vi "Dispatch Worker Mode Example(Async).vi"() -> ()   [LabVIEW 2014]
uses:
  user.lib/_NEVSTOP/JKI State Machine ++/_Support/JKISMQ/_JKISMQFGV.vi
  user.lib/_NEVSTOP/JKI State Machine ++/JKI-State-Machine-Plus.lvlib
panel:
  in  "Macro: Exit -@ Worker":bool
  in  "DoSth: DoA -@ Worker":bool
  in  "Name(\"\" to use uuid)":string="Event JKISM"
  out "State History":string
  in  "DoSth: DoA -> Worker":bool
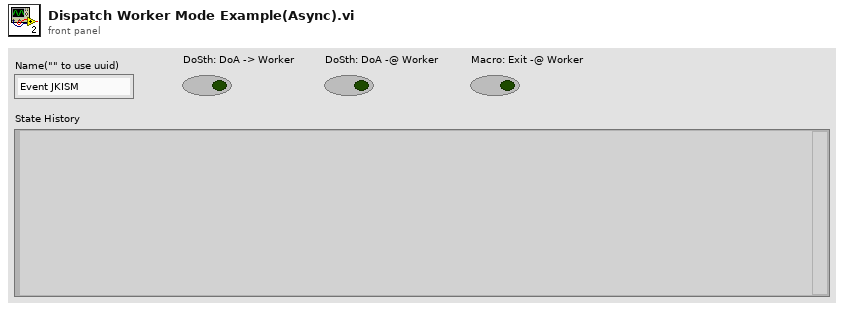
[diagram p1: front panel]
types:
  T1 = enum32{"Invalid", "Standard", "Closed", "Hidden", "Minimized", "Maximized"}
  T2 = enum32{"invalid app kind", "Development System", "Run Time System", "Student Edition", "Embedded LabVIEW", "Evaluation", "Custom"}
  T3 = cluster{"Core":cluster{"Current VI Reference":refnum<vi>, "Close Panel on Exit?":bool}, "Your Boolean data":bool, "Your string data":string}
  T4 = cluster{"Current VI Reference":refnum<vi>, "Close Panel on Exit?":bool}
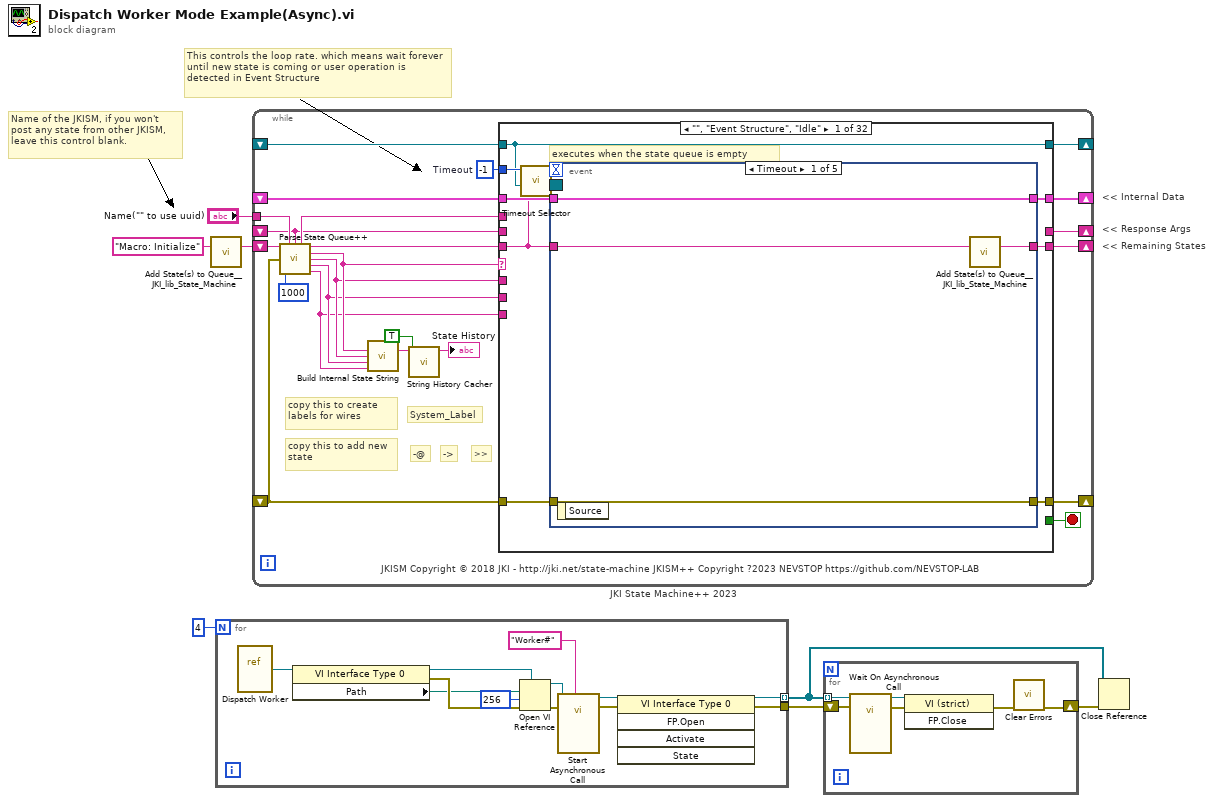
[diagram p0: block diagram]
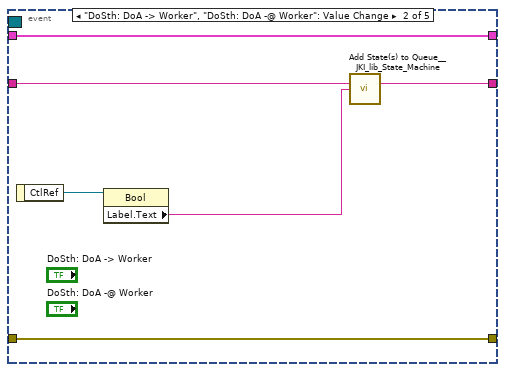
[diagram p2: hidden frame]
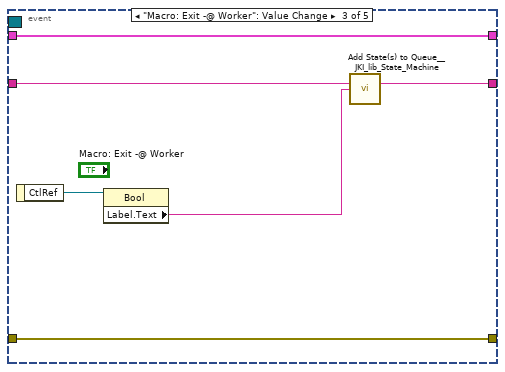
[diagram p3: hidden frame]
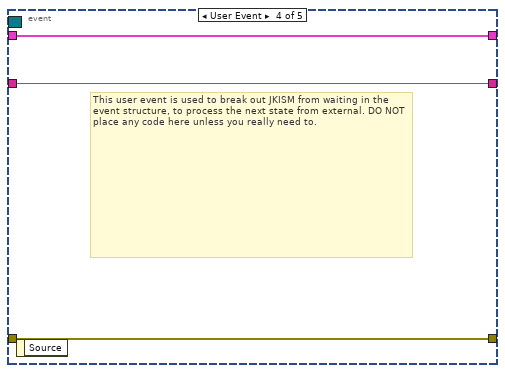
[diagram p4: hidden frame]
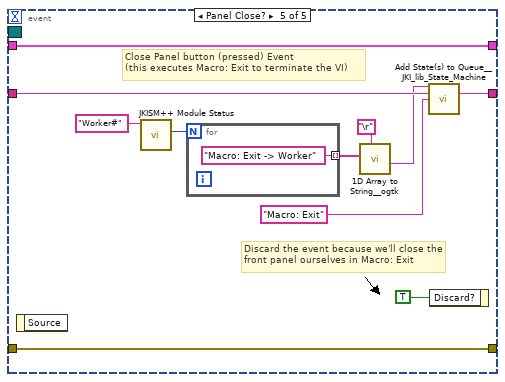
[diagram p5: hidden frame]
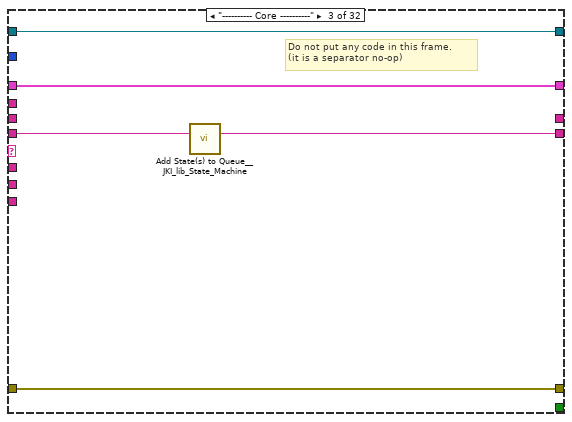
[diagram p7: hidden frame]
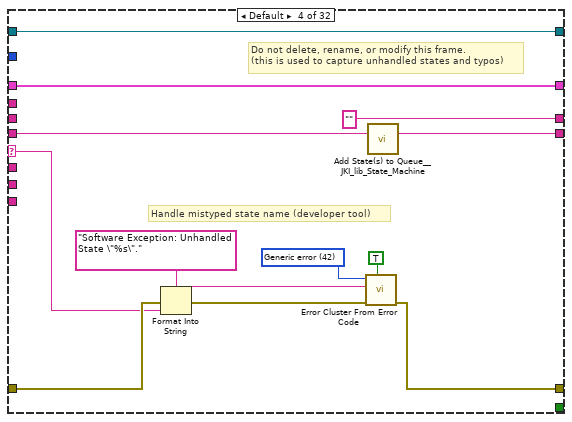
[diagram p8: hidden frame]
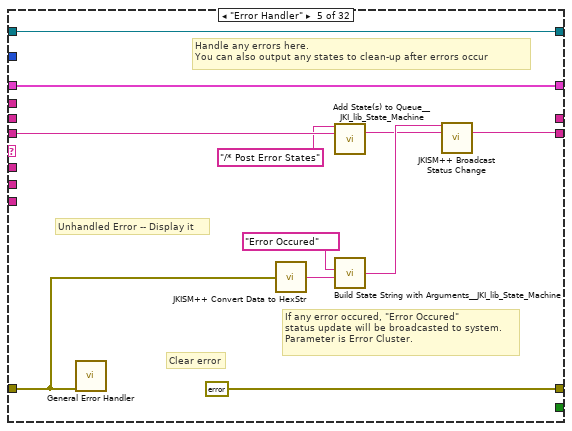
[diagram p9: hidden frame]
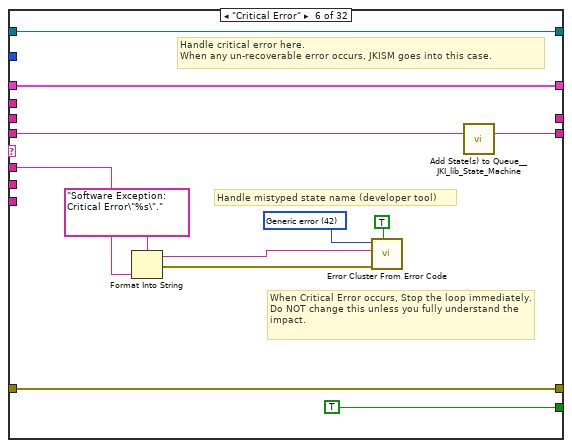
[diagram p10: hidden frame]
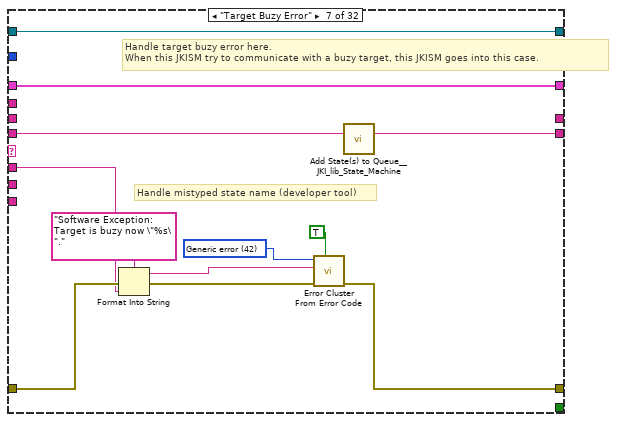
[diagram p11: hidden frame]
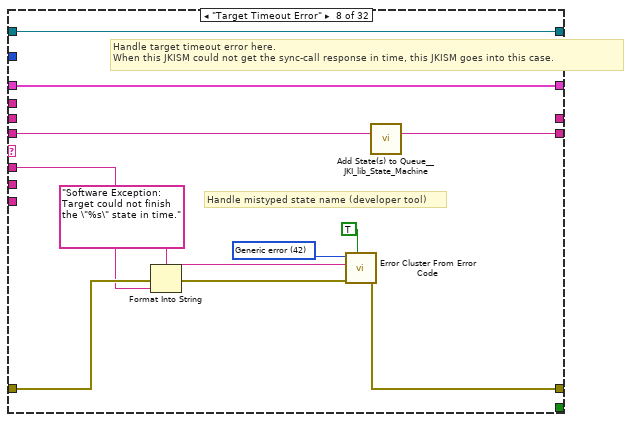
[diagram p12: hidden frame]
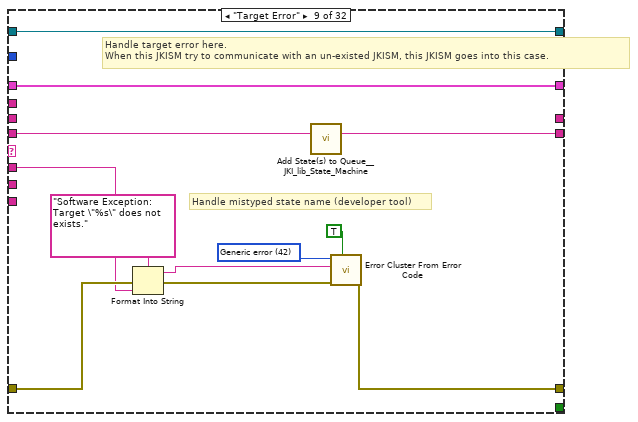
[diagram p13: hidden frame]
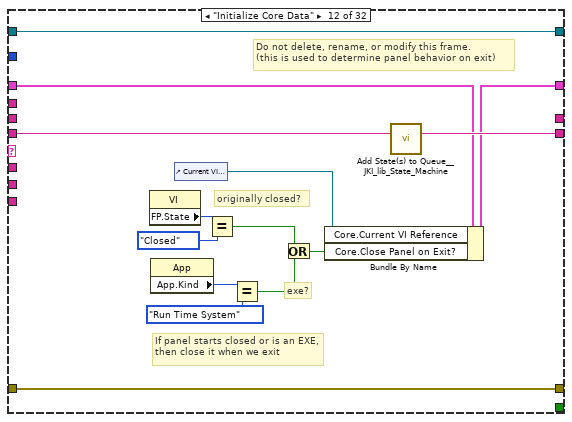
[diagram p16: hidden frame]
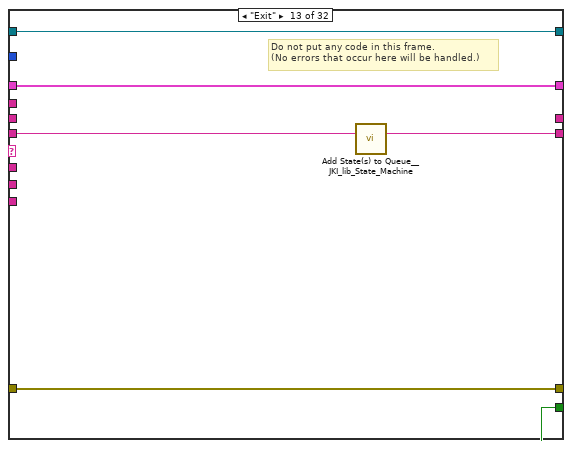
[diagram p17: hidden frame]
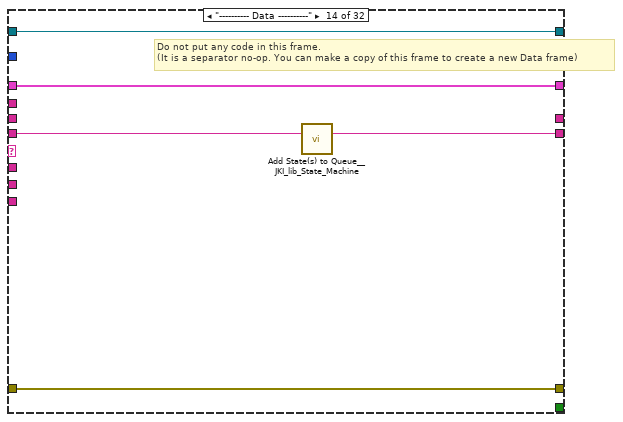
[diagram p18: hidden frame]
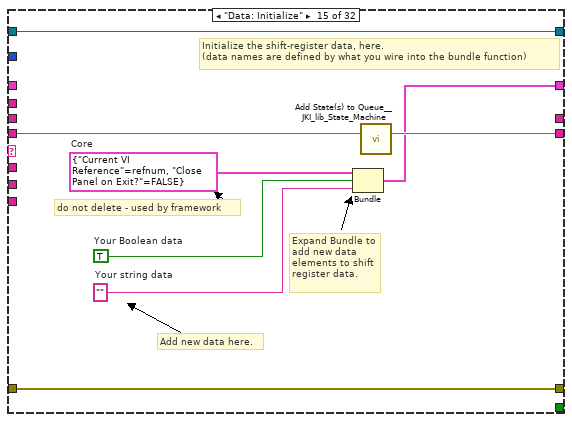
[diagram p19: hidden frame]
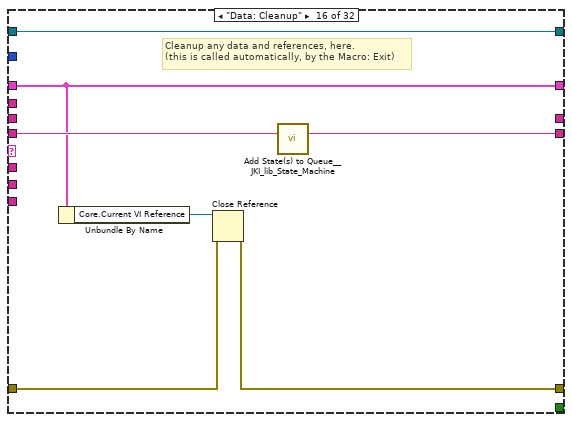
[diagram p20: hidden frame]
diagram:
  # "Name of the JKISM, if you won't post any state from other JKISM,  leave this control blank."
  # "This controls the loop rate. which means wait forever until new state is coming or user operation is detected in Event Structure"
  # "<< Internal Data"
  # "<< Response Args"
  # "<< Remaining States"
  n1 = call <vilib>:"Add State(s) to Queue__JKI_lib_State_Machine.vi"("State(s) in (\"\")"="Macro: Initialize") -> ("States Out"=w7:string)  [unwired: 14 in]
  n2 = for {
    N: 4 -> [_]
    tunnel: [w9] -> w4
    tunnel: [w10] -> w1 mode=indexing
    n3 = vi-ref "Dispatch Worker.vi"() -> (w13:refnum<vi>)
    n4 = property class="VI Interface Type 0"(reference=w13) -> (reference out=w17:refnum<vi>, error out=w15:errorcluster, "Path"=w14:path)  [unwired: 1 in]
    n5 = Open VI Reference(type specifier VI Refnum (for type only)=w17, vi path=w14, options=256, error in (no error)=w15) -> (vi reference=w16:refnum<vi>, error out=w12:errorcluster)  [unwired: 2 in]
    n6 = call-by-ref "Start Asynchronous Call"(reference=w16, error in=w12, "Name(\"\" to use uuid)"="Worker#" ("Name(\"\" to use uuid)")) -> (reference out=w11:refnum<vi>, error out=w8:errorcluster)  [unwired: 11 in]
    n7 = invoke class="VI Interface Type 0" method="FP.Open"(reference=w11, error in=w8) -> (reference out=w10:refnum<vi>, error out=w9:errorcluster)  [unwired: 3 in, 3 out]
  }
  n8 = while "JKI State Machine++ 2023" {
    shift-right: [w37] -> _
    shift-left: _ -> [w36]
    shift-right: [w40] -> _
    shift-left: _ -> [w34]
    shift-right: [w39] -> _
    shift-left: w7 -> [w41]
    tunnel: "Name(\"\" to use uuid)" -> [w29]
    shift-right: [w32] -> _
    shift-left: _ -> [w21]
    shift-right: [w31] -> _
    shift-left: _ -> [w30]
    stop <- w38 stop-if-true
    w35 = -1  # Timeout
    # "JKISM Copyright © 2018 JKI - http://jki.net/state-machine JKISM++ Copyright ?2023 NEVSTOP https://github.com/NEVSTOP-LAB"
    # "copy this to add new state"
    # ">>"
    # "->"
    # "-@"
    # "copy this to create labels for wires"
    # "System_Label"
    n9 = call "Parse State Queue++.vi"("State Queue"=w41, "Name(\"\" to use uuid)"=w29, "Response Arguments"=w21, "Error In (no error)"=w34, "Response Timeout(5000ms)"=1000 ("Response Timeout(1000ms)")) -> ("Name Used"=w22:string, "Remaining States"=w42:string, "Current State"=w26:string, "Arguments"=w25:string, "Argument - State"=w24:string, "From Who"=w23:string)  [unwired: 5 in]
    n10 = call "Build Internal State String.vi"("State"=w26, "Arguments (\"\")"=w25, "Arg-State (\"\")"=w24, "Source (\"\")"=w23) -> ("State with Arguments"=w27:string)  [unwired: 11 in]
    n11 = call "String History Cacher.vi"("Include Timestamp(F)"=TRUE, "String"=w27) -> ("String Cache"=→"State History":string)  [unwired: 9 in]
    n12 = case shown="\"\", \"Event Structure\", \"Idle\"" w26 {
      selector: w26 -> [_ _ _ w94 _ _ _ _ _ _ _ _ _ _ _ _ _ _ _ _ _ _ _ _ _ _ _ _ _ _ _ _]
      tunnel: w42 -> [w43 w85 w91 w98 w115 w125 w128 w145 w157 w166 w170 w185 w191 w196 w204 w211 w216 w222 w226 w232 w237 w244 w260 w330 w336 w347 w350 w355 w361 w369 w375 w381]
      tunnel: w25 -> [_ _ _ _ _ w118 w130 w141 w153 _ _ _ _ _ _ _ _ _ _ _ _ w239 w254 _ _ _ _ _ w358 _ _ _]
      tunnel: w36 -> [w50 w84 w88 w96 w113 w126 w132 w143 w155 w165 w169 w178 w189 w193 _ w206 w213 w221 w225 w229 w235 w242 w256 w327 w333 w344 w349 w354 w360 w366 w372 w378]
      tunnel: [w49 w86 w89 w100 errorcluster {"status"=FALSE, "code"=0, "source"=""} ("error out") w127 w135 w147 w159 w167 w171 w182 w188 w194 w201 w207 w214 w217 w224 w230 w234 w240 w257 w328 w334 w345 w351 w356 w362 w367 w373 w379] -> w40
      tunnel: w34 -> [w48 w86 w89 w99 w105 w127 w134 w146 w158 w167 w171 w182 w188 w194 w201 w208 w214 _ w227 w230 w234 w241 w258 w328 w334 w345 w351 w356 w362 w367 w373 w379]
      tunnel: [w51 w85 w90 w97 w106 w124 w133 w144 w156 w166 w170 w184 w190 w195 w203 w210 w215 w222 w226 w231 w236 w243 w259 w329 w335 w346 w350 w355 w361 w368 w374 w380] -> w39
      tunnel: [_ _ _ _ _ TRUE _ _ _ _ _ _ TRUE _ _ _ _ _ _ _ _ _ _ _ _ _ _ _ _ _ _ _] -> w38
      tunnel: [w47 w84 w88 w96 w113 w126 w132 w143 w155 w165 w169 w183 w189 w193 w202 w206 w213 w221 w225 w229 w235 w242 w256 w327 w333 w344 w349 w354 w360 w366 w372 w378] -> w37
      tunnel: w35 -> [w46 _ _ _ _ _ _ _ _ _ _ _ _ _ _ _ _ _ _ _ _ _ _ _ _ _ _ _ _ _ _ _]
      tunnel: w23 -> [_ _ _ _ _ _ _ _ _ _ _ _ _ _ _ _ _ _ _ _ _ _ _ _ _ _ _ _ _ _ _ _]
      tunnel: w24 -> [_ _ _ _ _ _ _ _ _ _ _ _ _ _ _ _ _ _ _ _ _ _ _ _ _ _ _ _ _ _ _ _]
      tunnel: [_ _ _ "" _ _ _ _ _ _ _ _ _ _ _ _ _ _ _ _ _ _ _ _ _ _ _ "API1 Response" w357 _ "DoA Finished" "DoB Finished"] -> w32
      tunnel: [w45 w83 w87 w92 w111 w116 w129 w140 w152 w164 w168 w172 w186 w192 w197 w205 w212 w220 w223 w228 w233 w238 w253 w326 w331 w337 w348 w353 w359 w365 w371 w377] -> w31
      tunnel: w30 -> [w45 w83 w87 w92 w111 w116 w129 w140 w152 w164 w168 w172 w186 w192 w197 w205 w212 _ w223 w228 w233 w238 w253 w326 w331 w337 w348 w353 w359 w365 w371 w377]
      tunnel: w22 -> [_ _ _ _ _ _ _ _ _ _ _ _ _ _ _ _ _ w219 _ _ _ _ _ _ _ _ _ _ _ _ _ _]
      tunnel: w21 -> [_ _ _ _ _ _ _ _ _ _ _ _ _ _ _ _ _ _ _ _ _ _ _ _ _ _ _ _ _ _ _ _]
      frame "", "Event Structure", "Idle" {
        # "executes when the state queue is empty"
        n13 = call "Timeout Selector.vi"("Remaining States"=w43, "Timeout Expected"=w46) -> ("Timeout"=w44:i32)  [unwired: 5 in]
        n14 = event shown="[0] Timeout" {
          selector: w45 -> [_ _ _ _ _]
          dyn-events: _ -> [_ _ _ _ _]
          timeout: w44 -> [_ _ _ _ _]
          tunnel: w43 -> [w55 w59 w65 w69 w81]
          tunnel: [w54 w58 w64 w69 w80] -> w51
          tunnel: w50 -> [w52 w60 w66 w70 w78]
          tunnel: [w53 w61 w67 w68 w79] -> w49
          tunnel: w48 -> [w53 w61 w67 w68 w79]
          tunnel: [w52 w60 w66 w70 w78] -> w47
          event Timeout {
            n15 = event-data() -> ()  [unwired: 1 in, 1 out]
            n16 = call <vilib>:"Add State(s) to Queue__JKI_lib_State_Machine.vi"("State(s) in (\"\")"=w55) -> ("States Out"=w54:string)  [unwired: 14 in]
          }
          event "DoSth: DoA -> Worker", "DoSth: DoA -@ Worker": Value Change {
            n17 = event-data() -> ("CtlRef"=w57:refnum<vi>)  [unwired: 1 in]
            n18 = property class="Bool"(reference=w57) -> ("Label.Text"=w56:string)  [unwired: 1 in, 2 out]
            n19 = call <vilib>:"Add State(s) to Queue__JKI_lib_State_Machine.vi"("State(s) in (\"\")"=w59, "State(s) at Back (\"\")"=w56) -> ("States Out"=w58:string)  [unwired: 13 in]
          }
          event "Macro: Exit -@ Worker": Value Change {
            n20 = event-data() -> ("CtlRef"=w63:refnum<vi>)  [unwired: 1 in]
            n21 = property class="Bool"(reference=w63) -> ("Label.Text"=w62:string)  [unwired: 1 in, 2 out]
            n22 = call <vilib>:"Add State(s) to Queue__JKI_lib_State_Machine.vi"("State(s) in (\"\")"=w65, "State(s) at Back (\"\")"=w62) -> ("States Out"=w64:string)  [unwired: 13 in]
          }
          event User Event {
            # "This user event is used to break out JKISM from waiting in the event structure, to process the next state from external. DO NOT place any code here unless you really need to."
            n23 = event-data() -> ()  [unwired: 1 in, 1 out]
          }
          event Panel Close? {
            # "Discard the event because we'll close the front panel ourselves in Macro: Exit"
            # "Close Panel button (pressed) Event\n(this executes Macro: Exit to terminate the VI)"
            n24 = event-data() -> ()  [unwired: 1 in, 1 out]
            n25 = call "JKISM++ Module Status.vi"("Name(\"\" to use uuid) in"="Worker#" ("Name(\"\" to use uuid)")) -> ("#AsWorker"=w76:i32)  [unwired: 7 in, 3 out]
            n26 = for {
              N: w76 -> [_]
              tunnel: ["Macro: Exit -> Worker"] -> w75 mode=indexing
            }
            n27 = call <userlib>:"1D Array to String__ogtk.vi"("delimiter (Tab)"="\r", "Array of Strings"=w75) -> ("delimited string"=w71:string)  [unwired: 9 in]
            n28 = call <vilib>:"Add State(s) to Queue__JKI_lib_State_Machine.vi"("State(s) in Front (\"\")"=w71, "State(s) in (\"\")"=w81, "State(s) at Back (\"\")"="Macro: Exit") -> ("States Out"=w80:string)  [unwired: 12 in]
            n29 = event-data("Discard?"=TRUE) -> ()  [unwired: 1 in, 1 out]
          }
        }
      }
      frame "JKISM++ Documentation" {
        # "JKISM++ Documentation"
        # "State Syntax:\nStateCategory: State >> Argument -@ JKISMName\nStateCategory: State >> Argument -> JKISMName\n\nLine Terminator: Line feed"
        # "Commenting:\nTo add a comment use \"//\" or \"#\" and all text to the right will be ignored\nCommenting Example:\nUI: Initialize // This initializes the UI\n# This whole line is a comment\n// Another comment line"
      }
      frame "---------- Core ----------" {
        # "Do not put any code in this frame.\n(it is a separator no-op)"
        n30 = call <vilib>:"Add State(s) to Queue__JKI_lib_State_Machine.vi"("State(s) in (\"\")"=w91) -> ("States Out"=w90:string)  [unwired: 14 in]
      }
      frame Default {
        w103 = 42 items=["No error", "Argument error", "Memory is full", "Out of zone", "End of file", "File already open", "Generic file I/O error", "File not found", "File permission error", "Disk is full", "Duplicate path", "Too many files open", "System feature not enabled", "Resource file not found", "Cannot add resource", "Resource not found", "Image not found", "Image memory error", "Pen does not exist", "Config type invalid", "Config token not found", "Config parse error", "Config memory error", "Bad external code format", "Bad external code offset", "External code not present", "Null window", "Destroy window error", "Null menu", "Print aborted", "Bad print record", "Print driver error", "Windows error during printing", "Memory error during printing", "Print dialog error", "Generic print error", "Invalid device refnum", "Device not found", "Device parameter error", "Device unit error", "Cannot open device", "Device call aborted", "Generic error", "Cancelled by user", "Object ID too low", "Object ID too high", "Object not in heap", "Unknown heap", "Unknown object (invalid DefProc)", "Unknown object (DefProc not in table)", "Message out of range", "Invalid (null) method", "Unknown message", "Manager call not supported", "Bad address", "Network operation in progress", "Network operation timed out", "Connection is busy", "Network attribute not supported", "Network error", "Address in use", "System out of memory", "Connection aborted", "Connection refused", "Not connected", "Already connected", "Connection closed", "Initialization error (interapplication manager)", "Bad occurrence", "Wait on unbound occurrence handler", "Occurrence queue overflow", "Datalog type conflict", "Unused", "Unrecognized type (interapplication manager)", "Memory corrupt", "Failed to make temporary DLL", "Old CIN version", "Drag socket not found", "Failed to load drop-object", "Failed to register OLE object", "Failed to release OLE object", "Format specifier type mismatch", "Unknown format specifier", "Too few format specifiers", "Too many format specifiers", "Scan failed", "Newer CIN version", "Error converting to variant", "Runtime menu error", "Password tampered", "Variant attribute not found", "Incompatible variant data type", "Event data is not available", "Event Store is not present", "Occurrence is not found", "Event Queue is not created", "Event info is not available", "Refnum passed is NULL", "Error retrieving Class GUID", "Error retrieving CoClass GUID", "Error retrieving TypeLib GUID.", "Bad built application magic bytes.", "Specific driver is different from the specific driver associated with the Logical Name.", "There is no session opened to the class driver.", "Max Error", "MAX - Error with config objects", "MAX - Error loading configuration", "MAX - Group not supported"]
        # "Do not delete, rename, or modify this frame.\n(this is used to capture unhandled states and typos)"
        # "Handle mistyped state name (developer tool)"
        n31 = Format Into String(format string="Software Exception: Unhandled State \"%s\"." ("message"), error in=w99, w94) -> (resulting string=w102:string, error out=w101:errorcluster)  [unwired: 1 in]
        n32 = call <vilib>:"Error Cluster From Error Code.vi"("show call chain? (False)"=TRUE, "error in (no error)"=w101, "error message (\"\")"=w102, "error code (0)"=w103) -> ("error out"=w100:errorcluster)  [unwired: 5 in]
        n33 = call <vilib>:"Add State(s) to Queue__JKI_lib_State_Machine.vi"("State(s) in (\"\")"=w98) -> ("States Out"=w97:string)  [unwired: 14 in]
      }
      frame "Error Handler" {
        # "If any error occured, \"Error Occured\" \nstatus update will be broadcasted to system.\nParameter is Error Cluster."
        # "Unhandled Error -- Display it"
        # "Handle any errors here.\nYou can also output any states to clean-up after errors occur"
        # "Clear error"
        n34 = call <vilib>:"General Error Handler.vi"("error in (no error)"=w105) -> ()  [unwired: 10 in, 5 out]
        n35 = call "JKISM++ Convert Data to HexStr.vi"("Variant"=w105) -> ("HEX String (0-9,A-F)"=w109:string)  [unwired: 8 in]
        n36 = call <vilib>:"Add State(s) to Queue__JKI_lib_State_Machine.vi"("State(s) in Front (\"\")"="/* Post Error States", "State(s) in (\"\")"=w115) -> ("States Out"=w107:string)  [unwired: 13 in]
        n37 = call <vilib>:"Build State String with Arguments__JKI_lib_State_Machine.vi"("Arguments (\"\")"=w109, "State"="Error Occured" ("Status with Arguments")) -> ("State with Arguments"=w108:string)  [unwired: 4 in]
        n38 = call "JKISM++ Broadcast Status Change.vi"("Status with Arguments"=w108, "State(s) in (\"\")"=w107) -> ("States Out"=w106:string)  [unwired: 13 in]
      }
      frame "Critical Error" {
        w122 = 42 items=["No error", "Argument error", "Memory is full", "Out of zone", "End of file", "File already open", "Generic file I/O error", "File not found", "File permission error", "Disk is full", "Duplicate path", "Too many files open", "System feature not enabled", "Resource file not found", "Cannot add resource", "Resource not found", "Image not found", "Image memory error", "Pen does not exist", "Config type invalid", "Config token not found", "Config parse error", "Config memory error", "Bad external code format", "Bad external code offset", "External code not present", "Null window", "Destroy window error", "Null menu", "Print aborted", "Bad print record", "Print driver error", "Windows error during printing", "Memory error during printing", "Print dialog error", "Generic print error", "Invalid device refnum", "Device not found", "Device parameter error", "Device unit error", "Cannot open device", "Device call aborted", "Generic error", "Cancelled by user", "Object ID too low", "Object ID too high", "Object not in heap", "Unknown heap", "Unknown object (invalid DefProc)", "Unknown object (DefProc not in table)", "Message out of range", "Invalid (null) method", "Unknown message", "Manager call not supported", "Bad address", "Network operation in progress", "Network operation timed out", "Connection is busy", "Network attribute not supported", "Network error", "Address in use", "System out of memory", "Connection aborted", "Connection refused", "Not connected", "Already connected", "Connection closed", "Initialization error (interapplication manager)", "Bad occurrence", "Wait on unbound occurrence handler", "Occurrence queue overflow", "Datalog type conflict", "Unused", "Unrecognized type (interapplication manager)", "Memory corrupt", "Failed to make temporary DLL", "Old CIN version", "Drag socket not found", "Failed to load drop-object", "Failed to register OLE object", "Failed to release OLE object", "Format specifier type mismatch", "Unknown format specifier", "Too few format specifiers", "Too many format specifiers", "Scan failed", "Newer CIN version", "Error converting to variant", "Runtime menu error", "Password tampered", "Variant attribute not found", "Incompatible variant data type", "Event data is not available", "Event Store is not present", "Occurrence is not found", "Event Queue is not created", "Event info is not available", "Refnum passed is NULL", "Error retrieving Class GUID", "Error retrieving CoClass GUID", "Error retrieving TypeLib GUID.", "Bad built application magic bytes.", "Specific driver is different from the specific driver associated with the Logical Name.", "There is no session opened to the class driver.", "Max Error", "MAX - Error with config objects", "MAX - Error loading configuration", "MAX - Group not supported"]
        # "Handle critical error here.\nWhen any un-recoverable error occurs, JKISM goes into this case."
        # "When Critical Error occurs, Stop the loop immediately. Do NOT change this unless you fully understand the impact."
        # "Handle mistyped state name (developer tool)"
        n39 = Format Into String(format string="Software Exception: Critical Error\"%s\"." ("message"), w118) -> (resulting string=w121:string, error out=w120:errorcluster)  [unwired: 2 in]
        n40 = call <vilib>:"Error Cluster From Error Code.vi"("show call chain? (False)"=TRUE, "error in (no error)"=w120, "error message (\"\")"=w121, "error code (0)"=w122) -> ()  [unwired: 5 in, 1 out]
        n41 = call <vilib>:"Add State(s) to Queue__JKI_lib_State_Machine.vi"("State(s) in (\"\")"=w125) -> ("States Out"=w124:string)  [unwired: 14 in]
      }
      frame "Target Buzy Error" {
        w138 = 42 items=["No error", "Argument error", "Memory is full", "Out of zone", "End of file", "File already open", "Generic file I/O error", "File not found", "File permission error", "Disk is full", "Duplicate path", "Too many files open", "System feature not enabled", "Resource file not found", "Cannot add resource", "Resource not found", "Image not found", "Image memory error", "Pen does not exist", "Config type invalid", "Config token not found", "Config parse error", "Config memory error", "Bad external code format", "Bad external code offset", "External code not present", "Null window", "Destroy window error", "Null menu", "Print aborted", "Bad print record", "Print driver error", "Windows error during printing", "Memory error during printing", "Print dialog error", "Generic print error", "Invalid device refnum", "Device not found", "Device parameter error", "Device unit error", "Cannot open device", "Device call aborted", "Generic error", "Cancelled by user", "Object ID too low", "Object ID too high", "Object not in heap", "Unknown heap", "Unknown object (invalid DefProc)", "Unknown object (DefProc not in table)", "Message out of range", "Invalid (null) method", "Unknown message", "Manager call not supported", "Bad address", "Network operation in progress", "Network operation timed out", "Connection is busy", "Network attribute not supported", "Network error", "Address in use", "System out of memory", "Connection aborted", "Connection refused", "Not connected", "Already connected", "Connection closed", "Initialization error (interapplication manager)", "Bad occurrence", "Wait on unbound occurrence handler", "Occurrence queue overflow", "Datalog type conflict", "Unused", "Unrecognized type (interapplication manager)", "Memory corrupt", "Failed to make temporary DLL", "Old CIN version", "Drag socket not found", "Failed to load drop-object", "Failed to register OLE object", "Failed to release OLE object", "Format specifier type mismatch", "Unknown format specifier", "Too few format specifiers", "Too many format specifiers", "Scan failed", "Newer CIN version", "Error converting to variant", "Runtime menu error", "Password tampered", "Variant attribute not found", "Incompatible variant data type", "Event data is not available", "Event Store is not present", "Occurrence is not found", "Event Queue is not created", "Event info is not available", "Refnum passed is NULL", "Error retrieving Class GUID", "Error retrieving CoClass GUID", "Error retrieving TypeLib GUID.", "Bad built application magic bytes.", "Specific driver is different from the specific driver associated with the Logical Name.", "There is no session opened to the class driver.", "Max Error", "MAX - Error with config objects", "MAX - Error loading configuration", "MAX - Group not supported"]
        # "Handle target buzy error here.\nWhen this JKISM try to communicate with a buzy target, this JKISM goes into this case."
        # "Handle mistyped state name (developer tool)"
        n42 = Format Into String(format string="Software Exception: Target is buzy now \"%s\"." ("message"), error in=w134, w130) -> (resulting string=w137:string, error out=w136:errorcluster)  [unwired: 1 in]
        n43 = call <vilib>:"Error Cluster From Error Code.vi"("show call chain? (False)"=TRUE, "error in (no error)"=w136, "error message (\"\")"=w137, "error code (0)"=w138) -> ("error out"=w135:errorcluster)  [unwired: 5 in]
        n44 = call <vilib>:"Add State(s) to Queue__JKI_lib_State_Machine.vi"("State(s) in (\"\")"=w128) -> ("States Out"=w133:string)  [unwired: 14 in]
      }
      frame "Target Timeout Error" {
        w150 = 42 items=["No error", "Argument error", "Memory is full", "Out of zone", "End of file", "File already open", "Generic file I/O error", "File not found", "File permission error", "Disk is full", "Duplicate path", "Too many files open", "System feature not enabled", "Resource file not found", "Cannot add resource", "Resource not found", "Image not found", "Image memory error", "Pen does not exist", "Config type invalid", "Config token not found", "Config parse error", "Config memory error", "Bad external code format", "Bad external code offset", "External code not present", "Null window", "Destroy window error", "Null menu", "Print aborted", "Bad print record", "Print driver error", "Windows error during printing", "Memory error during printing", "Print dialog error", "Generic print error", "Invalid device refnum", "Device not found", "Device parameter error", "Device unit error", "Cannot open device", "Device call aborted", "Generic error", "Cancelled by user", "Object ID too low", "Object ID too high", "Object not in heap", "Unknown heap", "Unknown object (invalid DefProc)", "Unknown object (DefProc not in table)", "Message out of range", "Invalid (null) method", "Unknown message", "Manager call not supported", "Bad address", "Network operation in progress", "Network operation timed out", "Connection is busy", "Network attribute not supported", "Network error", "Address in use", "System out of memory", "Connection aborted", "Connection refused", "Not connected", "Already connected", "Connection closed", "Initialization error (interapplication manager)", "Bad occurrence", "Wait on unbound occurrence handler", "Occurrence queue overflow", "Datalog type conflict", "Unused", "Unrecognized type (interapplication manager)", "Memory corrupt", "Failed to make temporary DLL", "Old CIN version", "Drag socket not found", "Failed to load drop-object", "Failed to register OLE object", "Failed to release OLE object", "Format specifier type mismatch", "Unknown format specifier", "Too few format specifiers", "Too many format specifiers", "Scan failed", "Newer CIN version", "Error converting to variant", "Runtime menu error", "Password tampered", "Variant attribute not found", "Incompatible variant data type", "Event data is not available", "Event Store is not present", "Occurrence is not found", "Event Queue is not created", "Event info is not available", "Refnum passed is NULL", "Error retrieving Class GUID", "Error retrieving CoClass GUID", "Error retrieving TypeLib GUID.", "Bad built application magic bytes.", "Specific driver is different from the specific driver associated with the Logical Name.", "There is no session opened to the class driver.", "Max Error", "MAX - Error with config objects", "MAX - Error loading configuration", "MAX - Group not supported"]
        # "Handle target timeout error here.\nWhen this JKISM could not get the sync-call response in time, this JKISM goes into this case."
        # "Handle mistyped state name (developer tool)"
        n45 = Format Into String(format string="Software Exception: Target could not finish the \"%s\" state in time." ("message"), error in=w146, w141) -> (resulting string=w149:string, error out=w148:errorcluster)  [unwired: 1 in]
        n46 = call <vilib>:"Error Cluster From Error Code.vi"("show call chain? (False)"=TRUE, "error in (no error)"=w148, "error message (\"\")"=w149, "error code (0)"=w150) -> ("error out"=w147:errorcluster)  [unwired: 5 in]
        n47 = call <vilib>:"Add State(s) to Queue__JKI_lib_State_Machine.vi"("State(s) in (\"\")"=w145) -> ("States Out"=w144:string)  [unwired: 14 in]
      }
      frame "Target Error" {
        w162 = 42 items=["No error", "Argument error", "Memory is full", "Out of zone", "End of file", "File already open", "Generic file I/O error", "File not found", "File permission error", "Disk is full", "Duplicate path", "Too many files open", "System feature not enabled", "Resource file not found", "Cannot add resource", "Resource not found", "Image not found", "Image memory error", "Pen does not exist", "Config type invalid", "Config token not found", "Config parse error", "Config memory error", "Bad external code format", "Bad external code offset", "External code not present", "Null window", "Destroy window error", "Null menu", "Print aborted", "Bad print record", "Print driver error", "Windows error during printing", "Memory error during printing", "Print dialog error", "Generic print error", "Invalid device refnum", "Device not found", "Device parameter error", "Device unit error", "Cannot open device", "Device call aborted", "Generic error", "Cancelled by user", "Object ID too low", "Object ID too high", "Object not in heap", "Unknown heap", "Unknown object (invalid DefProc)", "Unknown object (DefProc not in table)", "Message out of range", "Invalid (null) method", "Unknown message", "Manager call not supported", "Bad address", "Network operation in progress", "Network operation timed out", "Connection is busy", "Network attribute not supported", "Network error", "Address in use", "System out of memory", "Connection aborted", "Connection refused", "Not connected", "Already connected", "Connection closed", "Initialization error (interapplication manager)", "Bad occurrence", "Wait on unbound occurrence handler", "Occurrence queue overflow", "Datalog type conflict", "Unused", "Unrecognized type (interapplication manager)", "Memory corrupt", "Failed to make temporary DLL", "Old CIN version", "Drag socket not found", "Failed to load drop-object", "Failed to register OLE object", "Failed to release OLE object", "Format specifier type mismatch", "Unknown format specifier", "Too few format specifiers", "Too many format specifiers", "Scan failed", "Newer CIN version", "Error converting to variant", "Runtime menu error", "Password tampered", "Variant attribute not found", "Incompatible variant data type", "Event data is not available", "Event Store is not present", "Occurrence is not found", "Event Queue is not created", "Event info is not available", "Refnum passed is NULL", "Error retrieving Class GUID", "Error retrieving CoClass GUID", "Error retrieving TypeLib GUID.", "Bad built application magic bytes.", "Specific driver is different from the specific driver associated with the Logical Name.", "There is no session opened to the class driver.", "Max Error", "MAX - Error with config objects", "MAX - Error loading configuration", "MAX - Group not supported"]
        # "Handle target error here.\nWhen this JKISM try to communicate with an un-existed JKISM, this JKISM goes into this case."
        # "Handle mistyped state name (developer tool)"
        n48 = Format Into String(format string="Software Exception: Target \"%s\" does not exists." ("message"), error in=w158, w153) -> (resulting string=w161:string, error out=w160:errorcluster)  [unwired: 1 in]
        n49 = call <vilib>:"Add State(s) to Queue__JKI_lib_State_Machine.vi"("State(s) in (\"\")"=w157) -> ("States Out"=w156:string)  [unwired: 14 in]
        n50 = call <vilib>:"Error Cluster From Error Code.vi"("show call chain? (False)"=TRUE, "error in (no error)"=w160, "error message (\"\")"=w161, "error code (0)"=w162) -> ("error out"=w159:errorcluster)  [unwired: 5 in]
      }
      frame "Async Response", "Response" {
        # "Handle Async-call Response (\"Async Response\" for ->)"
        # "Handle Sync-call Response (\"Response\" for @)"
        # "After Message is excuted, JKISM+ goes to this state for recieve the response. \n    For Async Message(->), \"Async Response\" is used. This JKISM will goes to \"Async Message Posted\" immediately and recieve the \"Async Response\" after the callee finishes the message.\n    For Sync Message(@),  This JKISM will wait until the message is done and immidieatly goes to \"Response\""
      }
      frame "Async Message Posted" {
        # "Handle post action for async message (->)."
        # "After Async Message is posted (->), JKISM+ goes to this state for post-action. You can use Argument - State to tell which Async Message is called."
      }
      frame "Initialize Core Data" {
        # "Do not delete, rename, or modify this frame.\n(this is used to determine panel behavior on exit)"
        # "originally closed?"
        # "exe?"
        # "If panel starts closed or is an EXE, then close it when we exit"
        n51 = property class="VI"() -> ("FP.State"=w175:T1)  [unwired: 2 in, 2 out]
        n52 = property class="App"() -> ("App.Kind"=w181:T2)  [unwired: 2 in, 2 out]
        n53 = control-ref of="Current VI Reference"() -> (w176:refnum<vi>)
        n54 = Equal?(x=w175, y=T1."Closed" ("Front Panel Window:State")) -> (x = y?=w173:bool)
        n55 = Equal?(x=w181, y=T2."Run Time System" ("Application:Kind")) -> (x = y?=w179:bool)
        n56 = Or(x=w173, y=w179) -> (x .or. y?=w177:bool)
        n57 = Bundle By Name(cluster=w178, "Core.Current VI Reference"=w176, "Core.Close Panel on Exit?"=w177) -> (w183:T3)
        n58 = call <vilib>:"Add State(s) to Queue__JKI_lib_State_Machine.vi"("State(s) in (\"\")"=w185) -> ("States Out"=w184:string)  [unwired: 14 in]
      }
      frame "Exit" {
        # "Do not put any code in this frame.\n(No errors that occur here will be handled.)"
        n59 = call <vilib>:"Add State(s) to Queue__JKI_lib_State_Machine.vi"("State(s) in (\"\")"=w191) -> ("States Out"=w190:string)  [unwired: 14 in]
      }
      frame "---------- Data ----------" {
        # "Do not put any code in this frame.\n(It is a separator no-op. You can make a copy of this frame to create a new Data frame)"
        n60 = call <vilib>:"Add State(s) to Queue__JKI_lib_State_Machine.vi"("State(s) in (\"\")"=w196) -> ("States Out"=w195:string)  [unwired: 14 in]
      }
      frame "Data: Initialize" {
        w198 = T4 {"Current VI Reference"=refnum, "Close Panel on Exit?"=FALSE}  # Core
        w200 = TRUE  # Your Boolean data
        w199 = ""  # Your string data
        # "do not delete - used by framework"
        # "Expand Bundle to add new data elements to shift register data."
        # "Add new data here."
        # "Initialize the shift-register data, here.\n(data names are defined by what you wire into the bundle function)"
        n61 = Bundle("Core"=w198, "Your Boolean data"=w200, "Your string data"=w199) -> (w202:T3)  [unwired: 1 in]
        n62 = call <vilib>:"Add State(s) to Queue__JKI_lib_State_Machine.vi"("State(s) in (\"\")"=w204) -> ("States Out"=w203:string)  [unwired: 14 in]
      }
      frame "Data: Cleanup" {
        # "Cleanup any data and references, here.\n(this is called automatically, by the Macro: Exit)"
        n63 = Unbundle By Name(w206) -> ("Core.Current VI Reference"=w209:refnum<vi>)
        n64 = Close Reference(reference=w209, error in (no error)=w208) -> (error out=w207:errorcluster)
        n65 = call <vilib>:"Add State(s) to Queue__JKI_lib_State_Machine.vi"("State(s) in (\"\")"=w211) -> ("States Out"=w210:string)  [unwired: 14 in]
      }
      frame "---------- Events ----------" {
        # "Do not put any code in this frame.\n(It is a separator no-op. You can make a copy of this frame to create a new UI frame)"
        n66 = call <vilib>:"Add State(s) to Queue__JKI_lib_State_Machine.vi"("State(s) in (\"\")"=w216) -> ("States Out"=w215:string)  [unwired: 14 in]
      }
      frame "Events: Register" {
        # "Register message event to break Waiting in Event structure."
        n67 = call "JKISM++ Get New State Notifier Event.vi"("Name(\"\" to use uuid) in"=w219) -> ("Error out"=w217:errorcluster, "New State Notifier Event"=w218:refnum<user-event>)  [unwired: 9 in]
        n68 = register-events(w218) -> (reference out=w220:refnum<event-registration>)  [unwired: 2 in, 1 out]
      }
      frame "Events: Unregister" {
        n69 = Unregister For Events(event registration refnum=w223, error in=w227) -> (error out=w224:errorcluster)
      }
      frame "---------- UI ----------" {
        # "Do not put any code in this frame.\n(It is a separator no-op. You can make a copy of this frame to create a new UI frame)"
        n70 = call <vilib>:"Add State(s) to Queue__JKI_lib_State_Machine.vi"("State(s) in (\"\")"=w232) -> ("States Out"=w231:string)  [unwired: 14 in]
      }
      frame "UI: Initialize" {
        # "Initialize the User Interface, here.\n(this is called automatically, by the Macro: Init)"
        n71 = call <vilib>:"Add State(s) to Queue__JKI_lib_State_Machine.vi"("State(s) in (\"\")"=w237) -> ("States Out"=w236:string)  [unwired: 14 in]
      }
      frame "UI: Cursor Set" {
        # "Argument"
        # "Set and Unset Cursor Busy.\n(Usage: \"UI: Cursor Set >> Busy|Idle\")"
        n72 = disable-structure shown="TARGET_TYPE!=Windows" {
          disable-tunnel: w241 -> [w247 w252]
          disable-tunnel: [w246 w252] -> w240
          disable-tunnel: w239 -> [w245 _]
          frame condition #0 (active) {
            n73 = case shown="\"Idle\", Default" w245 {
              tunnel: w247 -> [w249 w251]
              tunnel: [w248 w250] -> w246
              frame "Idle", Default {
                n74 = call <vilib>:"Unset Busy.vi"("error in (no error)"=w249) -> ("error out"=w248:errorcluster)  [unwired: 10 in]
              }
              frame "Busy" {
                n75 = call <vilib>:"Set Busy.vi"("error in (no error)"=w251) -> ("error out"=w250:errorcluster)  [unwired: 9 in, 1 out]
              }
            }
          }
          frame condition #1 {
          }
        }
        n76 = call <vilib>:"Add State(s) to Queue__JKI_lib_State_Machine.vi"("State(s) in (\"\")"=w244) -> ("States Out"=w243:string)  [unwired: 14 in]
      }
      frame "UI: Front Panel State" {
        # "Argument"
        # "Set Front Panel Open or Closed\n(Usage: \"UI: Front Panel State >> Open|Close\")"
        n77 = Unbundle By Name(w256) -> ("Core.Current VI Reference"=w255:refnum<vi>)
        n78 = call <vilib>:"Add State(s) to Queue__JKI_lib_State_Machine.vi"("State(s) in (\"\")"=w260) -> ("States Out"=w259:string)  [unwired: 14 in]
        n79 = case shown="\"Minimize\", \"Minimized\"" w254 {
          tunnel: w258 -> [w266 w281 w292 w305 w318]
          tunnel: [w268 w282 w294 w307 w320] -> w257
          tunnel: w255 -> [w267 w279 w293 w306 w319]
          frame "Open", "Standard", Default {
            w261 = T1."Standard" ("State")
            n80 = property class="VI"(reference=w267, error in=w266) -> (reference out=w264:refnum<vi>, error out=w265:errorcluster, "FP.State"=w263:T1)
            n81 = Not Equal?(x=w263, y=w261) -> (x != y?=w262:bool)
            n82 = case shown="True" w262 {
              tunnel: [w272 w274] -> w268
              tunnel: w265 -> [w271 w274]
              tunnel: w264 -> [w270 _]
              tunnel: w261 -> [w269 _]
              frame True {
                n83 = invoke class="VI" method="FP.Open"(reference=w270, error in=w271, "Activate"=TRUE, "State"=w269) -> (error out=w272:errorcluster)  [unwired: 1 in, 4 out]
              }
              frame False {
              }
            }
          }
          frame "Close", "Closed" {
            n84 = property class="VI"(reference=w279, error in=w281) -> (reference out=w278:refnum<vi>, error out=w280:errorcluster, "FP.State"=w276:T1)
            n85 = Not Equal?(x=w276, y=T1."Closed" ("Front Panel Window:State")) -> (x != y?=w275:bool)
            n86 = case shown="True" w275 {
              tunnel: [w283 w286] -> w282
              tunnel: w280 -> [w283 w285]
              tunnel: w278 -> [_ w284]
              frame False {
              }
              frame True {
                n87 = invoke class="VI" method="FP.Close"(reference=w284, error in=w285) -> (error out=w286:errorcluster)  [unwired: 1 in, 2 out]
              }
            }
          }
          frame "Hidden", "Hide" {
            w287 = T1."Hidden" ("State")
            n88 = property class="VI"(reference=w293, error in=w292) -> (reference out=w290:refnum<vi>, error out=w291:errorcluster, "FP.State"=w289:T1)
            n89 = Not Equal?(x=w289, y=w287) -> (x != y?=w288:bool)
            n90 = case shown="True" w288 {
              tunnel: [w298 w299] -> w294
              tunnel: w291 -> [w297 w299]
              tunnel: w290 -> [w296 _]
              tunnel: w287 -> [w295 _]
              frame True {
                n91 = invoke class="VI" method="FP.Open"(reference=w296, error in=w297, "State"=w295) -> (error out=w298:errorcluster)  [unwired: 2 in, 4 out]
              }
              frame False {
              }
            }
          }
          frame "Minimize", "Minimized" {
            w300 = T1."Minimized" ("State")
            n92 = property class="VI"(reference=w306, error in=w305) -> (reference out=w303:refnum<vi>, error out=w304:errorcluster, "FP.State"=w302:T1)
            n93 = Not Equal?(x=w302, y=w300) -> (x != y?=w301:bool)
            n94 = case shown="True" w301 {
              tunnel: [w311 w312] -> w307
              tunnel: w304 -> [w310 w312]
              tunnel: w303 -> [w309 _]
              tunnel: w300 -> [w308 _]
              frame True {
                n95 = invoke class="VI" method="FP.Open"(reference=w309, error in=w310, "State"=w308) -> (error out=w311:errorcluster)  [unwired: 2 in, 4 out]
              }
              frame False {
              }
            }
          }
          frame "Maximize", "Maximized" {
            w313 = T1."Maximized" ("State")
            n96 = property class="VI"(reference=w319, error in=w318) -> (reference out=w316:refnum<vi>, error out=w317:errorcluster, "FP.State"=w315:T1)
            n97 = Not Equal?(x=w315, y=w313) -> (x != y?=w314:bool)
            n98 = case shown="True" w314 {
              tunnel: [w324 w325] -> w320
              tunnel: w317 -> [w323 w325]
              tunnel: w316 -> [w322 _]
              tunnel: w313 -> [w321 _]
              frame True {
                n99 = invoke class="VI" method="FP.Open"(reference=w322, error in=w323, "State"=w321) -> (error out=w324:errorcluster)  [unwired: 2 in, 4 out]
              }
              frame False {
              }
            }
          }
        }
      }
      frame "---------- Macro ----------" {
        # "Do not put any code in this frame.\n(It is a separator no-op. You can make a copy of this frame to create a new Macro frame)"
        n100 = call <vilib>:"Add State(s) to Queue__JKI_lib_State_Machine.vi"("State(s) in (\"\")"=w330) -> ("States Out"=w329:string)  [unwired: 14 in]
      }
      frame "Macro: Initialize" {
        w332 = "Data: Initialize\nInitialize Core Data\nEvents: Register\nUI: Initialize\nUI: Front Panel State >> Open"  # Data: Initialize Initialize Core Data Events: Register UI: Initialize UI: Front Panel State >> Open
        # "Initialization Macro\n(This is called once, when the VI starts)"
        n101 = call <vilib>:"Add State(s) to Queue__JKI_lib_State_Machine.vi"("State(s) in Front (\"\")"=w332, "State(s) in (\"\")"=w336) -> ("States Out"=w335:string)  [unwired: 13 in]
      }
      frame "Macro: Exit" {
        # "Exit Macro\n(This is called once, when the VI exits)"
        n102 = Unbundle By Name(w344) -> ("Core.Close Panel on Exit?"=w343:bool)
        n103 = Select(t="UI: Front Panel State >> Close", s=w343, f="") -> (s? t:f=w340:string)
        n104 = call <vilib>:"Add State(s) to Queue__JKI_lib_State_Machine.vi"("State(s) in (\"\")"=w340, "State(s) at Back (\"\")"="Data: Cleanup\nEvents: Unregister\nExit") -> ("States Out"=w338:string)  [unwired: 13 in]
        n105 = call <vilib>:"Add State(s) to Queue__JKI_lib_State_Machine.vi"("State(s) in Front (\"\")"=w338, "State(s) in (\"\")"=w347) -> ("States Out"=w346:string)  [unwired: 13 in]
      }
      frame "---------- API ----------" {
        # "Do not put any code in this frame.\n(It is a separator no-op. This category is recommanded to use for external API)"
      }
      frame "API: API1" {
        # "If you need to tell who triggered this state , use this string. If it's this case itself, this string is \"\"."
        # "Deal with the parameter if any"
        # "Connect this to return the response of your API"
        # "Copy/Rename this case for your own API"
      }
      frame "API: API2" {
        # "unpack HexStr  to Variant\nif complex parameter is needed."
        # "Copy/Rename this case for your own API"
        n106 = call "JKISM++ Convert HexStr to Data.vi"("HEX String"=w358) -> ()  [unwired: 8 in, 1 out]
        n107 = disable-structure shown="Disabled" {
          disable-tunnel: [w363 "API2 Response"] -> w357
          frame Disabled {
            # "pack variant to hexstr \nif complex response is needed."
            # "complex Response"
            n108 = call "JKISM++ Convert Data to HexStr.vi"() -> ("HEX String (0-9,A-F)"=w363:string)  [unwired: 9 in]
          }
          frame Enabled {
          }
        }
      }
      frame "---------- DoSth ----------" {
        # "Template Separator\n(You can make a copy of, or modify, this frame)"
        n109 = call <vilib>:"Add State(s) to Queue__JKI_lib_State_Machine.vi"("State(s) in (\"\")"=w369) -> ("States Out"=w368:string)  [unwired: 14 in]
      }
      frame "DoSth: DoA" {
        # "Your code here.\n(You can make a copy of, or modify, this frame)"
        n110 = call <vilib>:"Add State(s) to Queue__JKI_lib_State_Machine.vi"("State(s) in (\"\")"=w375) -> ("States Out"=w374:string)  [unwired: 14 in]
      }
      frame "DoSth: DoB" {
        # "Your code here.\n(You can make a copy of, or modify, this frame)"
        n111 = call <vilib>:"Add State(s) to Queue__JKI_lib_State_Machine.vi"("State(s) in (\"\")"=w381) -> ("States Out"=w380:string)  [unwired: 14 in]
      }
    }
  }
  n112 = for {
    shift-right: [w382] -> w3
    shift-left: w4 -> [w387]
    tunnel: w1 -> [w386] mode=indexing
    n113 = call-by-ref "Wait On Asynchronous Call"(reference=w386, error in=w387) -> (reference out=w385:refnum<vi>, error out=w383:errorcluster)  [unwired: 12 in]
    n114 = invoke class="VI (strict)" method="FP.Close"(reference=w385, error in=w383) -> (error out=w384:errorcluster)  [unwired: 1 in, 2 out]
    n115 = call <vilib>:"Clear Errors.vi"("error in (no error)"=w384) -> ("error out"=w382:errorcluster)  [unwired: 5 in, 1 out]
  }
  n116 = Close Reference(reference=w1, error in (no error)=w3) -> ()  [unwired: 1 out]
